vi "note bounds.vi"(9 "Note Polygon":cluster{"x":i16, "y":i16}[](array[cluster])=[{"x"=10, "y"=0}, {"x"=23, "y"=0}, {"x"=23, "y"=150}, {"x"=0, "y"=150}, {"x"=0, "y"=100}, {"x"=10, "y"=100}, {"x"=10, "y"=0}], 11 "Anticlockwise rotations [0-3] (0)":i32) -> (2 "Bounds":cluster{"Max":i16, "Min":i16})   [LabVIEW 2020, in "midi-ui.lvclass"]
uses:
  midi-ui.lvclass
  midi-ui.lvclass/midi-ui.ctl
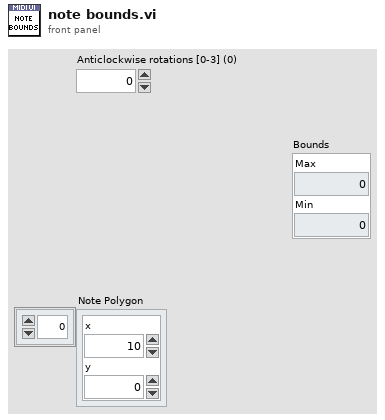
[diagram p1: front panel]
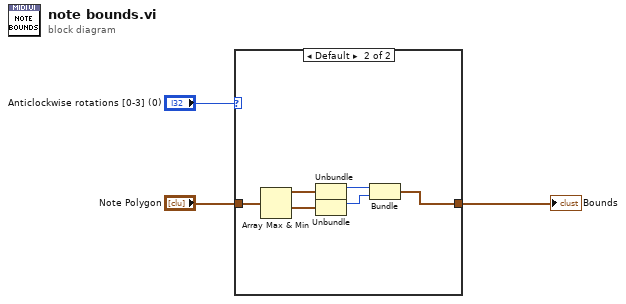
[diagram p0: block diagram]
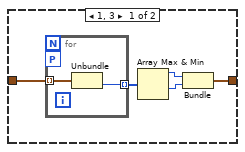
[diagram p2: hidden frame]
diagram:
  n1 = case shown="Default" "Anticlockwise rotations [0-3] (0)" {
    tunnel: "Note Polygon" -> [w8 w16]
    tunnel: [w4 w11] -> w1
    frame 1, 3 {
      n2 = for {
        tunnel: w8 -> [w10] mode=indexing
        tunnel: [w9] -> w7 mode=indexing
        workers-P: _ -> [_]
        n3 = Unbundle(w10) -> ("y"=w9:i16)  [unwired: 1 out]
      }
      n4 = Array Max & Min(array=w7) -> (max value=w6:i16, min value=w5:i16)  [unwired: 2 out]
      n5 = Bundle(w6, w5) -> (w4:cluster{i16, i16})  [unwired: 1 in]
    }
    frame Default {
      n6 = Array Max & Min(array=w16) -> (max value=w14:cluster{"x":i16, "y":i16}, min value=w15:cluster{"x":i16, "y":i16})  [unwired: 2 out]
      n7 = Unbundle(w14) -> ("x"=w13:i16)  [unwired: 1 out]
      n8 = Unbundle(w15) -> ("x"=w12:i16)  [unwired: 1 out]
      n9 = Bundle("x"=w13, "x"=w12) -> (w11:cluster{"x":i16, "x":i16})  [unwired: 1 in]
    }
  }
  "Bounds" <- w1
